vi "DriveEN.vi"() -> (1 "AxisError":i32, 2 "DriveError":i16, 3 "DoCancleErrorStatus":bool)   [LabVIEW 2011]
panel:
  out "DoCancleError":errorcluster
  out "error out":errorcluster
  out "AAABuild":i32
  in  "MintController":refnum<k7>(container)
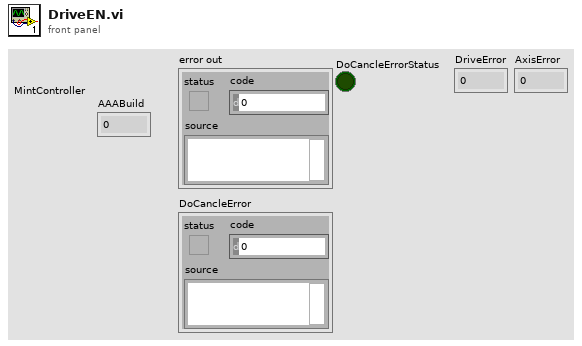
[diagram p1: front panel]
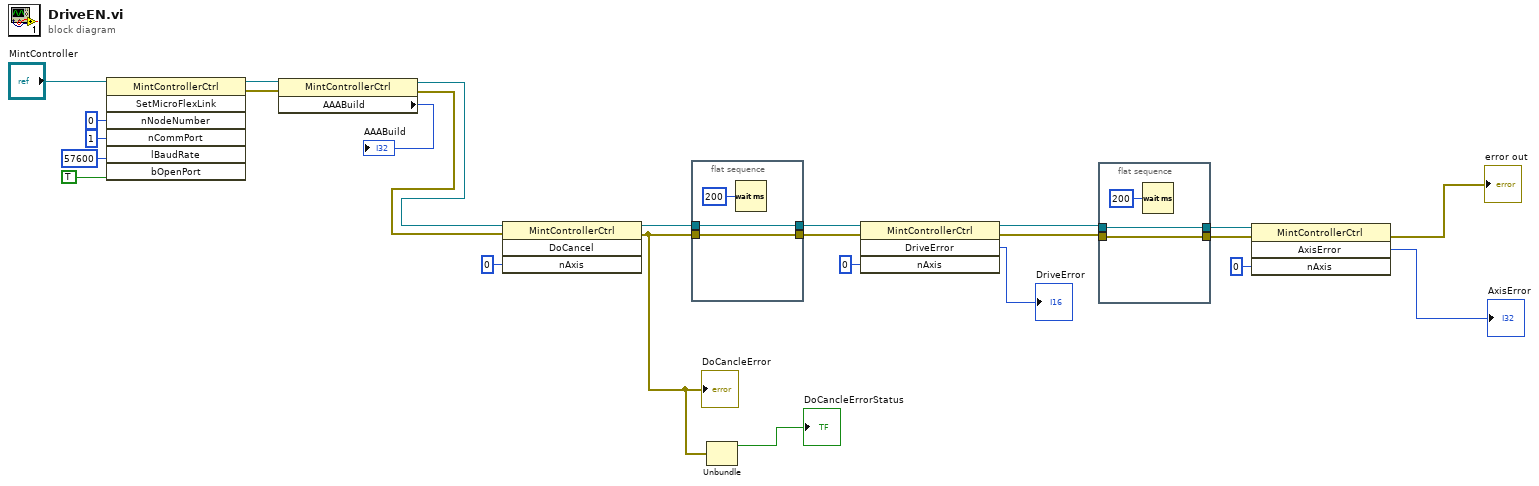
[diagram p0: block diagram]
diagram:
  n1 = invoke class="MintControllerCtrl" method="SetMicroFlexLink"(reference="MintController", "nNodeNumber"=i16 0, "nCommPort"=i16 1, "lBaudRate"=57600, "bOpenPort"=TRUE) -> (reference out=w25:refnum<k7>, error out=w19:errorcluster)  [unwired: 2 in, 5 out]
  n2 = property class="MintControllerCtrl"(reference=w25, error in=w19) -> (reference out=w16:refnum<k7>, error out=w15:errorcluster, "AAABuild"=→"AAABuild":i32)
  n3 = invoke class="MintControllerCtrl" method="DoCancel"(reference=w16, error in=w15, "nAxis"=i16 0) -> (reference out=w8:refnum<k7>, error out=w2:errorcluster)  [unwired: 1 in, 2 out]
  "DoCancleError" <- w2
  n4 = flat-sequence {
    tunnel: [w28] -> w9
    tunnel: w8 -> [w28]
    tunnel: w2 -> [w27]
    tunnel: [w27] -> w7
    frame #0 {
      n5 = Wait (ms)(milliseconds to wait=u32 200) -> ()  [unwired: 1 out]
    }
  }
  n6 = Unbundle(w2) -> ("status"=→"DoCancleErrorStatus":bool)  [unwired: 2 out]
  n7 = invoke class="MintControllerCtrl" method="DriveError"(reference=w9, error in=w7, "nAxis"=i16 0) -> (reference out=w6:refnum<k7>, error out=w5:errorcluster, "DriveError"=→"DriveError":i16)  [unwired: 1 in, 1 out]
  n8 = flat-sequence {
    tunnel: [w31] -> w4
    tunnel: w6 -> [w31]
    tunnel: w5 -> [w30]
    tunnel: [w30] -> w3
    frame #0 {
      n9 = Wait (ms)(milliseconds to wait=u32 200) -> ()  [unwired: 1 out]
    }
  }
  n10 = invoke class="MintControllerCtrl" method="AxisError"(reference=w4, error in=w3, "nAxis"=i16 0) -> (error out=→"error out":errorcluster, "AxisError"=→"AxisError":i32)  [unwired: 1 in, 2 out]
